vi "Enable Reference Channel.vi"(8 "error in (no error)":errorcluster {"code" format="%.0x"}, 9 "Channel Enabled (True)":bool=TRUE, 10 "Reference Channel (\"REF1\")":string(combo)="REF1", 11 "VISA Resource Name":refnum<visa-resource-name>) -> (0 "error out":errorcluster {"code" format="%.0x"}, 3 "VISA Resource Name Out":refnum<visa-resource-name>)   [LabVIEW 2010, in "Tektronix TDS 3000 Series.lvlib"]
doc: "This VI enables or disables a reference channel\n\nNotes:\n\n(1) You can enable a reference channel only after you store a waveform to the reference channel. Use the tktds3k Store Wfm To Reference Channel VIs to a store waveform to a reference channel.\n\n(2) Disabling a reference channel does not clear the waveform that you stored in that reference channel."
uses:
  <instrlib>/Tektronix TDS 3000 Series/Tektronix TDS 3000 Series.lvlib
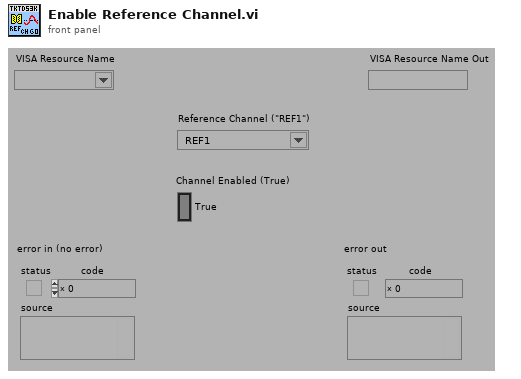
[diagram p1: front panel]
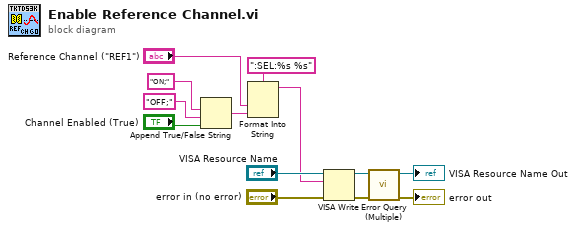
[diagram p0: block diagram]
diagram:
  n1 = Append True/False String(1:"Channel Enabled (True)", 2:"OFF;" ("false string"), 3:"ON;" ("true string")) -> (0:w8:string)  [unwired: 1 in]
  n2 = Format Into String(format string=":SEL:%s %s", "Reference Channel (\"REF1\")", w8) -> (resulting string=w5:string)  [unwired: 2 in, 1 out]
  n3 = VISA Write(VISA resource name="VISA Resource Name", write buffer=w5, error in (no error)="error in (no error)") -> (VISA resource name out=w4:refnum<visa-resource-name>, error out=w3:errorcluster)  [unwired: 1 out]
  n4 = call <instrlib>:"Error Query (Multiple).vi"("error in (no error)"=w3, "VISA Resource Name"=w4) -> ("error out"=→"error out":errorcluster, "VISA Resource Name Out"=→"VISA Resource Name Out":refnum<visa-resource-name>)  [unwired: 6 in, 2 out]
